vi "Change sequence player data file.vi"(4 "Other path":path) -> (1 "File path out":path)   [LabVIEW 2016]
doc: "Select the acquisition directory which contains the sequence to be used."
uses:
  GLIMPSE Globals.vi
panel:
  in  "Selection":i32(listbox)
  in  "Cancel":bool
  in  "OK":bool
  out "Highest number path":path
  out "Last used path":path
  # "Last used\nHighest number\nOther"
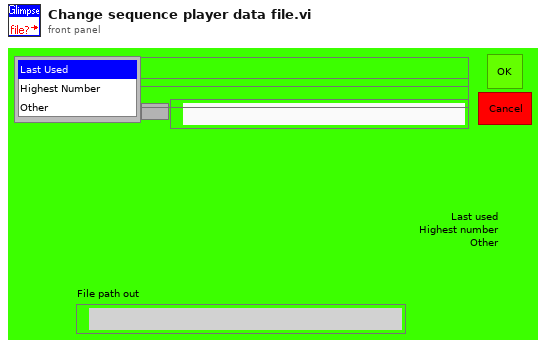
[diagram p1: front panel]
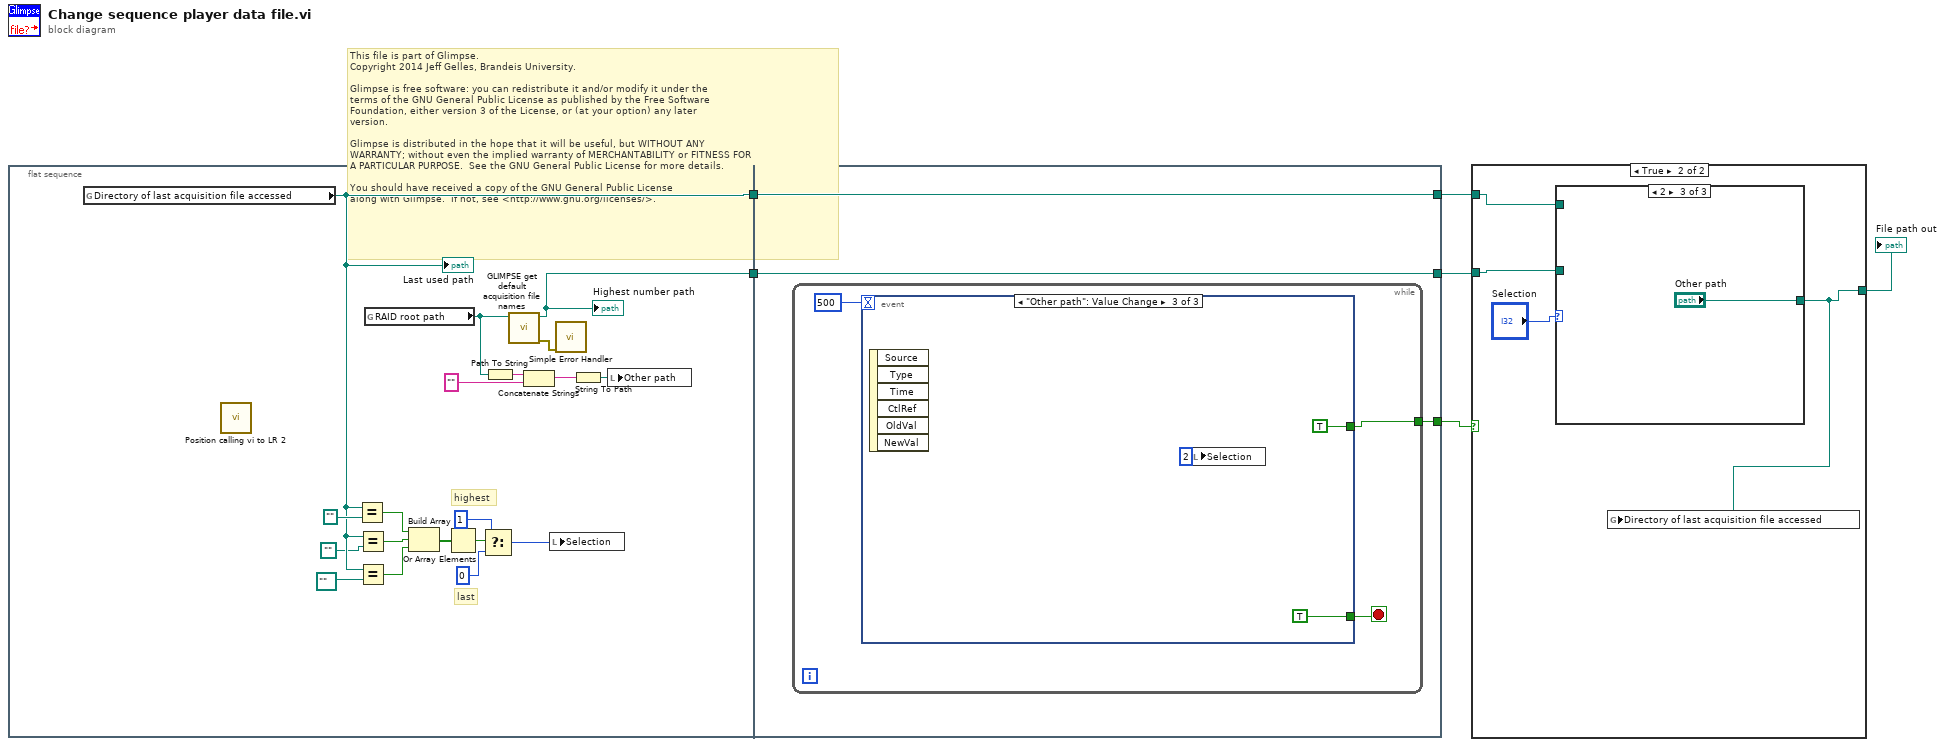
[diagram p0: block diagram]
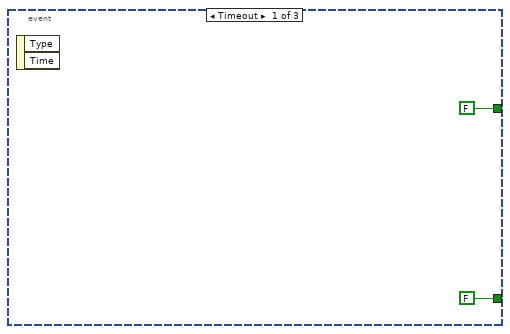
[diagram p2: hidden frame]
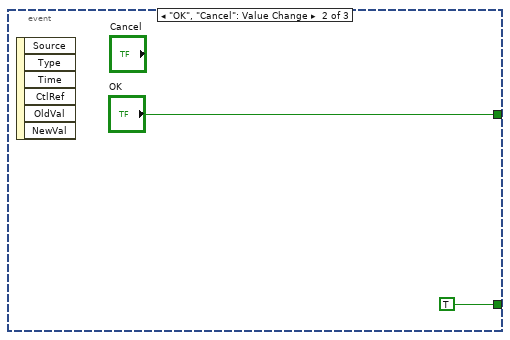
[diagram p3: hidden frame]
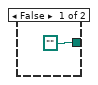
[diagram p4: hidden frame]
diagram:
  # "This file is part of Glimpse. \nCopyright 2014 Jeff Gelles, Brandeis University.    \n\nGlimpse is free software: you can redistribute it and/or modify it under the \nterms of the GNU General Public License as published by the Free Software \nFoundation, either version 3 of the License, or (at your option) any later \nversion.\n\nGlimpse is distributed in the hope that it will be useful, but WITHOUT ANY \nWARRANTY; without even the implied warranty of MERCHANTABILITY or FITNESS FOR \nA PARTICULAR PURPOSE.  See the GNU General Public License for more details.\n\nYou should have received a copy of the GNU General Public License\nalong with Glimpse.  If not, see <http://www.gnu.org/licenses/>."
  n1 = flat-sequence {
    tunnel: [w13] -> w3
    tunnel: [w24] -> w2
    tunnel: [w28] -> w5
    tunnel: w3 -> [w28]
    tunnel: [w27] -> w4
    tunnel: w2 -> [w27]
    tunnel: [w26] -> w1
    frame #0 {
      # "last"
      # "highest"
      n2 = global read "GLIMPSE Globals.vi" "Directory of last acquisition file accessed"() -> (w13:path)
      "Last used path" <- w13
      n3 = call "Position calling vi to LR 2.vi"() -> ()  [unwired: 2 in, 4 out]
      n4 = Equal?(x=w13, y=path "") -> (x = y?=w16:bool)
      n5 = Equal?(x=w13, y=path "") -> (x = y?=w15:bool)
      n6 = Equal?(x=w13, y=path "") -> (x = y?=w14:bool)
      n7 = global read "GLIMPSE Globals.vi" "RAID root path"() -> (w23:path)
      n8 = Build Array(w16, w15, w14) -> (w17:bool[])
      n9 = Or Array Elements(Boolean array=w17) -> (logical OR=w10:bool)
      n10 = Select(t=1, s=w10, f=0 ("t")) -> (s? t:f=w9:i32)
      n11 = Path To String(path=w23) -> (string=w20:string)
      n12 = call "GLIMPSE get default acquisition file names.vi"("RAID root path"=w23) -> ("error out"=w25:errorcluster, "last directory path"=w24:path)  [unwired: 1 in, 6 out]
      "Highest number path" <- w24
      n13 = Concatenate Strings(w20, "" ("string")) -> (w21:string)
      n14 = local write "Selection"(w9) -> ()
      n15 = call <vilib>:"Simple Error Handler.vi"("error in (no error)"=w25) -> ()  [unwired: 1 in, 8 out]
      n16 = String To Path(string=w21) -> (path=w19:path)
      n17 = local write "Other path"(w19) -> ()
    }
    frame #1 {
      n18 = while {
        tunnel: [w29] -> w26
        stop <- w30 stop-if-true
        n19 = event shown="[2] \"Other path\": Value Change" {
          selector: _ -> [_ _ _]
          dyn-events: _ -> [_ _ _]
          timeout: 500 -> [_ _ _]
          tunnel: [FALSE TRUE TRUE] -> w30
          tunnel: [FALSE ("OK") "OK" TRUE ("OK")] -> w29
          event Timeout {
            n20 = event-data() -> ()  [unwired: 3 out]
          }
          event "OK", "Cancel": Value Change {
            n21 = event-data() -> ()  [unwired: 7 out]
          }
          event "Other path": Value Change {
            n22 = event-data() -> ()  [unwired: 7 out]
            n23 = local write "Selection"(2 ("Selection")) -> ()
          }
        }
      }
    }
  }
  n24 = case shown="True" w1 {
    tunnel: [path "" w41] -> w6
    tunnel: w5 -> [_ w43]
    tunnel: w4 -> [_ w42]
    frame False {
    }
    frame True {
      n25 = case shown="2" "Selection" {
        tunnel: [w44 w45 "Other path"] -> w41
        tunnel: w43 -> [w44 _ _]
        tunnel: w42 -> [_ w45 _]
        frame 0, Default {
          # "last"
        }
        frame 1 {
          # "highest"
        }
        frame 2 {
        }
      }
      n26 = global write "GLIMPSE Globals.vi" "Directory of last acquisition file accessed"(w41) -> ()
    }
  }
  "File path out" <- w6
